vi "Set Windows Size.vi"(4 "Position":cluster{"X":i32, "Y":i32}, 6 "Size":cluster{"cx":i32, "cy":i32}, 8 "error in (no error)":errorcluster, 9 "uFlags":u32(ring)=1 items=["SWP_ASYNCWINDOWPOS"=16384, "SWP_DEFERERASE"=8192, "SWP_DRAWFRAME"=32, "SWP_HIDEWINDOW"=128, "SWP_NOACTIVATE"=16, "SWP_NOCOPYBITS"=256, "SWP_NOMOVE"=2, "SWP_NOOWNERZORDER"=512, "SWP_NOREDRAW"=8, "SWP_NOSENDCHANGING"=1024, "SWP_NOSIZE"=1, "SWP_NOZORDER"=4, "SWP_SHOWWINDOW"=64], 10 "hWndInsertAfter":string(combo), 11 "hWnd":i32) -> (0 "error out":errorcluster, 3 "hWnd out":i32)   [LabVIEW 2019]
uses:
  user32.dll
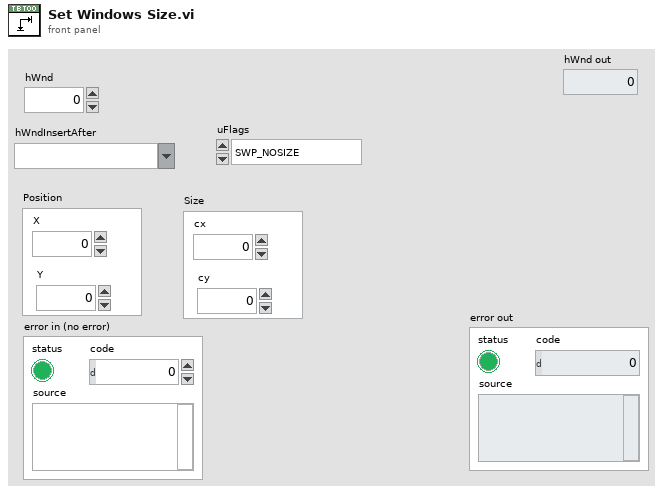
[diagram p1: front panel]
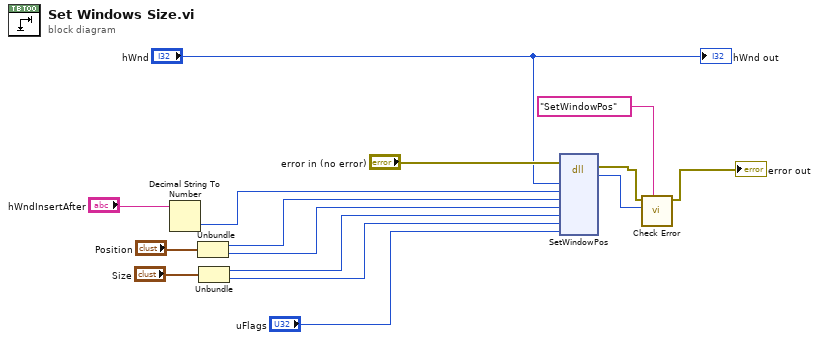
[diagram p0: block diagram]
diagram:
  n1 = Decimal String To Number(string="hWndInsertAfter") -> (number=w7:i32)  [unwired: 2 in, 1 out]
  n2 = Unbundle("Position") -> ("X"=w13:i32, "Y"=w12:i32)
  n3 = Unbundle("Size") -> ("cx"=w10:i32, "cy"=w9:i32)
  n4 = dll-call lib="USER32.DLL" fn="SetWindowPos"(error in="error in (no error)", "hWnd"="hWnd", "hWndInsertAfter"=w7, "left"=w13, "top"=w12, "width"=w10, "height"=w9, "fuFlags"="uFlags") -> (error out=w4:errorcluster, "error"=w2:i32)  [unwired: 9 in, 1 out]
  n5 = call "Check Error.vi"("Description"="SetWindowPos", "Return Code"=w2, "error in (no error)"=w4) -> ("error out"=→"error out":errorcluster)  [unwired: 8 in]
  "hWnd out" <- "hWnd"
